vi "NI MAX (BR) (1).vi"() -> ()   [LabVIEW 2025]
panel:
  out "Boolean 3":bool
  out "Boolean 2":bool
  out "Boolean":bool
  out "Numeric 4":dbl
  in  "Numeric 2":dbl
  in  "Numeric":dbl
  in  "String":string
  in  "s":dbl
  out "Numeric 3":dbl
  in  "b":dbl
  in  "a":dbl
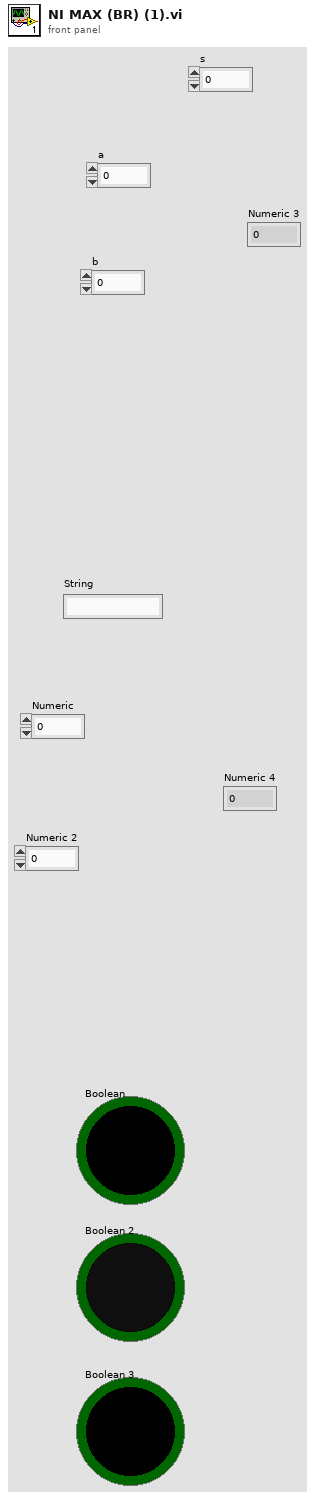
[diagram p1: front panel]
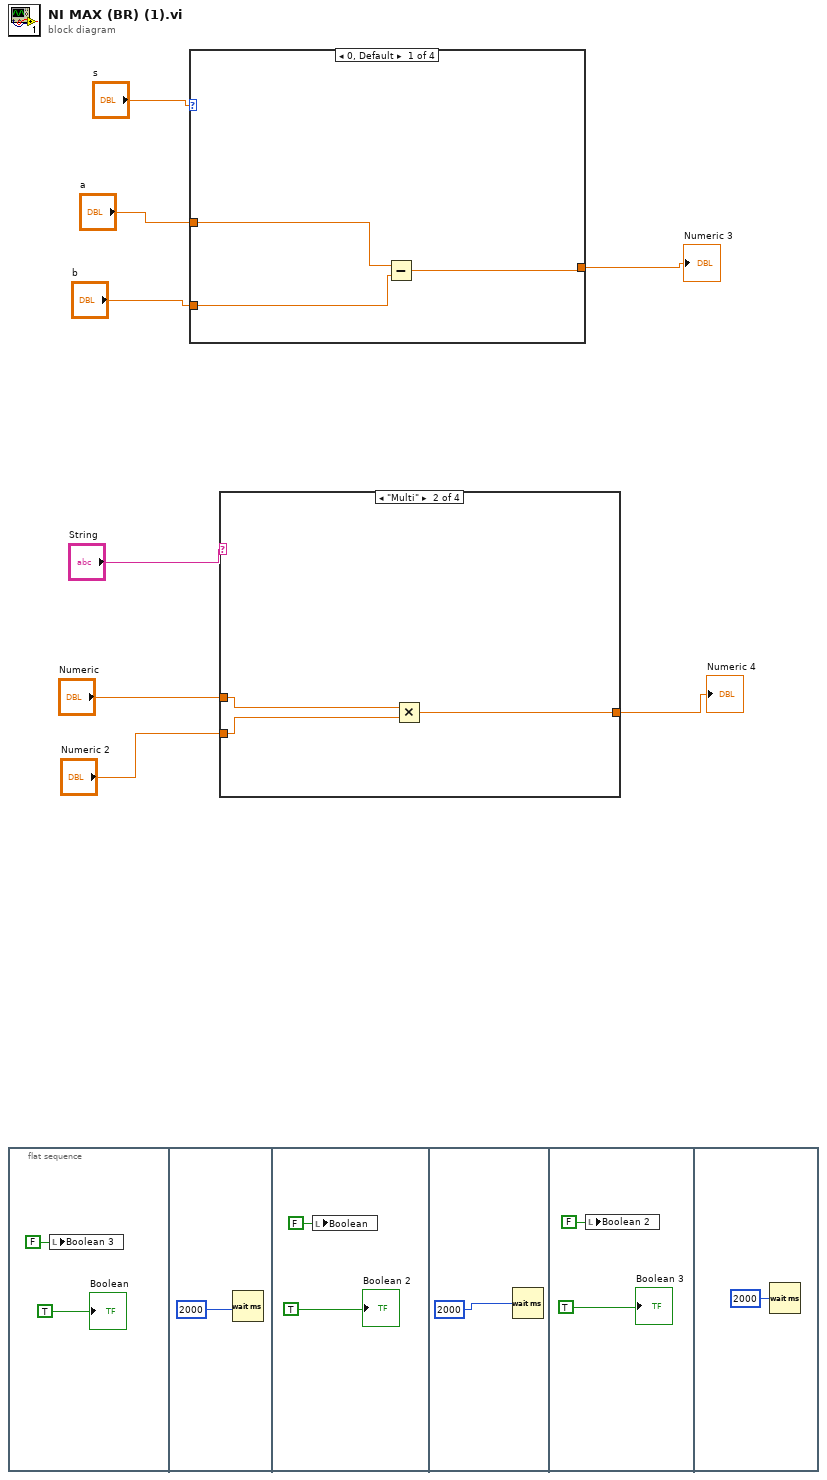
[diagram p0: block diagram]
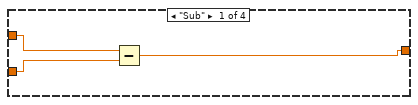
[diagram p2: hidden frame]
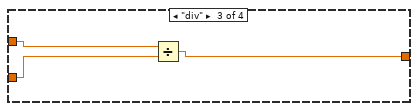
[diagram p3: hidden frame]
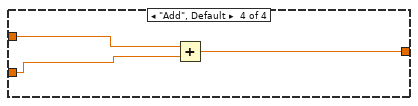
[diagram p4: hidden frame]
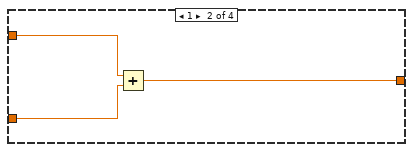
[diagram p5: hidden frame]
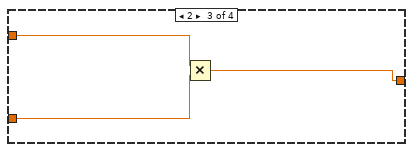
[diagram p6: hidden frame]
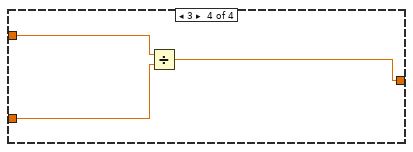
[diagram p7: hidden frame]
diagram:
  n1 = flat-sequence {
    frame #0 {
      n2 = local write "Boolean 3"(FALSE ("Boolean 3")) -> ()
      "Boolean" <- TRUE ("Boolean")
    }
    frame #1 {
      n3 = Wait (ms)(milliseconds to wait=u32 2000) -> ()  [unwired: 1 out]
    }
    frame #2 {
      n4 = local write "Boolean"(FALSE ("Boolean")) -> ()
      "Boolean 2" <- TRUE ("Boolean 2")
    }
    frame #3 {
      n5 = Wait (ms)(milliseconds to wait=u32 2000 ("millisecond timer value")) -> ()  [unwired: 1 out]
    }
    frame #4 {
      n6 = local write "Boolean 2"(FALSE ("Boolean 2")) -> ()
      "Boolean 3" <- TRUE ("Boolean 3")
    }
    frame #5 {
      n7 = Wait (ms)(milliseconds to wait=u32 2000) -> ()  [unwired: 1 out]
    }
  }
  n8 = case shown="0, Default" "s" {
    tunnel: "a" -> [w18 w23 w26 w29]
    tunnel: "b" -> [w19 w22 w25 w28]
    tunnel: [w20 w21 w24 w27] -> w6
    frame 0, Default {
      n9 = Subtract(x=w18, y=w19) -> (x-y=w20:dbl)
    }
    frame 1 {
      n10 = Add(x=w23, y=w22) -> (x+y=w21:dbl)
    }
    frame 2 {
      n11 = Multiply(x=w26, y=w25) -> (x*y=w24:dbl)
    }
    frame 3 {
      n12 = Divide(x=w29, y=w28) -> (x/y=w27:dbl)
    }
  }
  "Numeric 3" <- w6
  n13 = case shown="\"Multi\"" "String" {
    tunnel: "Numeric" -> [w32 w35 w38 w41]
    tunnel: "Numeric 2" -> [w31 w34 w37 w40]
    tunnel: [w30 w33 w36 w39] -> w1
    frame "Sub" {
      n14 = Subtract(x=w32, y=w31) -> (x-y=w30:dbl)
    }
    frame "Multi" {
      n15 = Multiply(x=w35, y=w34) -> (x*y=w33:dbl)
    }
    frame "div" {
      n16 = Divide(x=w38, y=w37) -> (x/y=w36:dbl)
    }
    frame "Add", Default {
      n17 = Add(x=w41, y=w40) -> (x+y=w39:dbl)
    }
  }
  "Numeric 4" <- w1
